vi "speed.vi"(5 "speed":dbl=5.0, 6 "dt Scaling":dbl=0.5, 7 "input":path, 9 "replacementString":string="Speed.wav") -> (4 "output":path)   [LabVIEW 2012]
uses:
  <vilib>/addons/Time Frequency Analysis/Transform.llb/TFA Online Gabor Transform (Real).vi
  <vilib>/addons/Time Frequency Analysis/Transform.llb/TFA Online Gabor Expansion (Real).vi
  <vilib>/Analysis/2dsp.llb/Resample (constant to constant,single -channel).vi
  <vilib>/addons/_Advanced Signal Processing/NI_AdvSigProcTFA.lvlib
  <vilib>/Analysis/NI_AALPro.lvlib
panel:
  out "Waveform Graph 2":waveform(dbl)(graph)
  out "Waveform Graph":waveform(dbl)(graph)
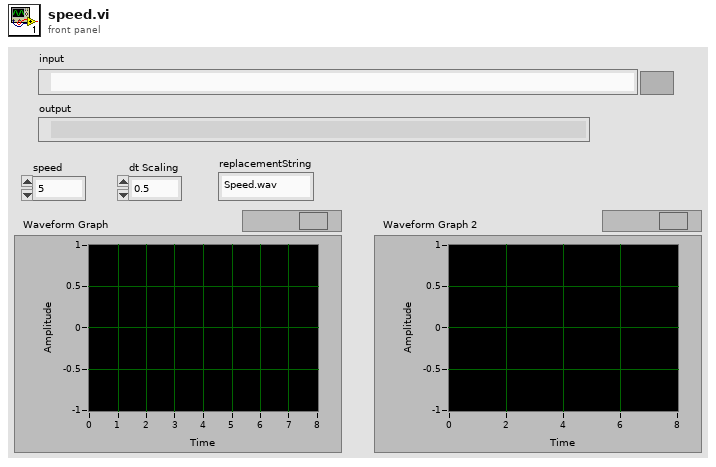
[diagram p1: front panel]
types:
  T1 = cluster{"synthesis window":dbl[], "dM (time steps)":i32, "N (frequency bins)":i32}
  T2 = cluster{"analysis window":dbl[], "dM (time steps)":i32, "N (frequency bins)":i32}
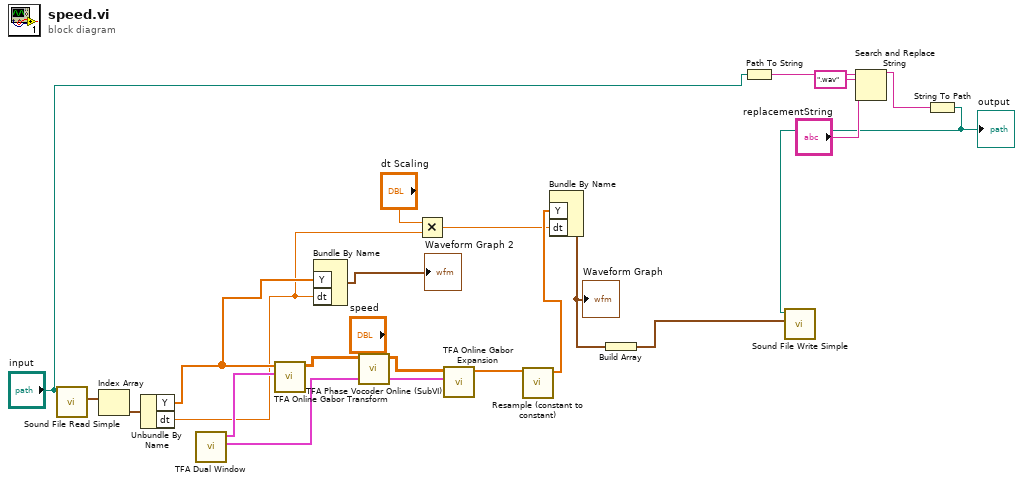
[diagram p0: block diagram]
diagram:
  n1 = call <vilib>:"Sound File Read Simple.vi"("path"="input") -> ("data"=w21:waveform(dbl)[])  [unwired: 7 in, 3 out]
  n2 = Index Array(array=w21) -> (element=w22:waveform(dbl))  [unwired: 1 in]
  n3 = Unbundle By Name(w22) -> ("Y"=w15:dbl[], "dt"=w9:dbl)
  n4 = call <vilib>:"TFA Dual Window.vi"() -> ("synthesis info"=w19:T1, "analysis info"=w20:T2)  [unwired: 4 in, 6 out]
  n5 = call-poly <vilib>:"TFA Online Gabor Transform.vi"("transform info"=w20, "signal"=w15) -> ("Gabor coef"=w18:cdb[][])  [unwired: 2 in, 7 out]
  n6 = Bundle By Name("Y"=w15, "dt"=w9) -> (→"Waveform Graph 2":waveform(dbl))  [unwired: 1 in]
  n7 = call "TFA Phase Vocoder Online (SubVI).vi"("squeeze"="speed", "STFT coef in"=w18) -> ("STFT coef out"=w16:cdb[][])  [unwired: 2 in, 7 out]
  n8 = Multiply(x="dt Scaling", y=w9) -> (x*y=w10:dbl)
  n9 = call-poly <vilib>:"TFA Online Gabor Expansion.vi"("expansion info"=w19, "Gabor coef"=w16) -> ("signal"=w17:dbl[])  [unwired: 1 in, 8 out]
  n10 = call-poly <vilib>:"Resample (constant to constant).vi"("X"=w17) -> ("Y"=w14:dbl[])  [unwired: 6 in, 4 out]
  n11 = Bundle By Name("Y"=w14, "dt"=w10) -> (w13:waveform(dbl))  [unwired: 1 in]
  "Waveform Graph" <- w13
  n12 = Build Array(w13) -> (w12:waveform(dbl)[])
  n13 = Path To String(path="input") -> (string=w1:string)
  n14 = Search and Replace String(input string=w1, search string=".wav", replace string="replacementString") -> (result string=w4:string)  [unwired: 5 in, 3 out]
  n15 = String To Path(string=w4) -> (path=w3:path)
  "output" <- w3
  n16 = call <vilib>:"Sound File Write Simple.vi"("data"=w12, "path"=w3) -> ()  [unwired: 8 in, 2 out]
